vi "Get IRP Waveform.vi"(10 "Channel config":T2={"Voltage channel index"=1, "Shunt channel index"=2, "Shunt resistance"=10.0}, 11 "array":waveform(dbl)[](array[waveform])) -> (1 "Power waveform out":waveform(dbl), 2 "Resistance waveform out":waveform(dbl), 3 "Current waveform out":waveform(dbl), 4 "Channel names":T1)   [LabVIEW 2019]
doc: "This example demonstrates how to acquire a continuous amount of data (Waveform) using the DAQ device's internal clock. It also shows how to synchronize two devices for different device families (E Series, S Series, M Series, X Series, DSA, and SC Express), to simultaneously acquire the data.\n\nFor instructions on how to connect your signals to the DAQ device, refer to your device documentation."
panel:
  # "Get IRP Waveform"
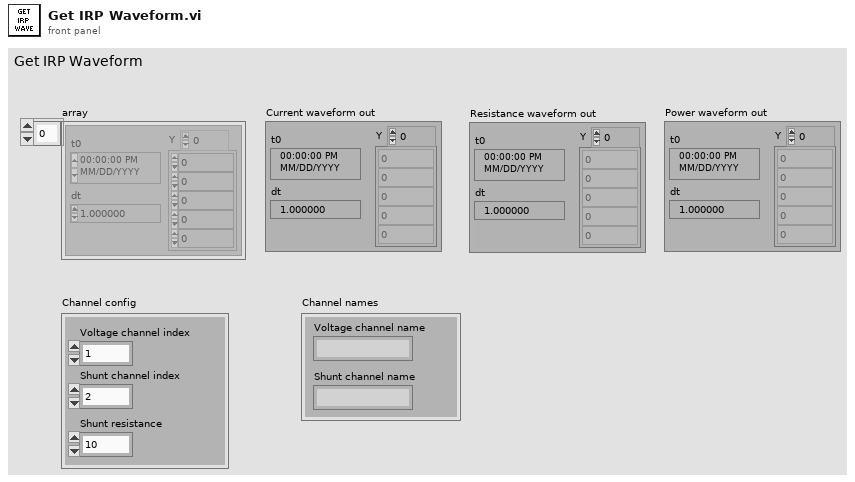
[diagram p1: front panel]
types:
  T1 = cluster{"Voltage channel name":string, "Shunt channel name":string}
  T2 = cluster{"Voltage channel index":i32, "Shunt channel index":i32, "Shunt resistance":dbl}
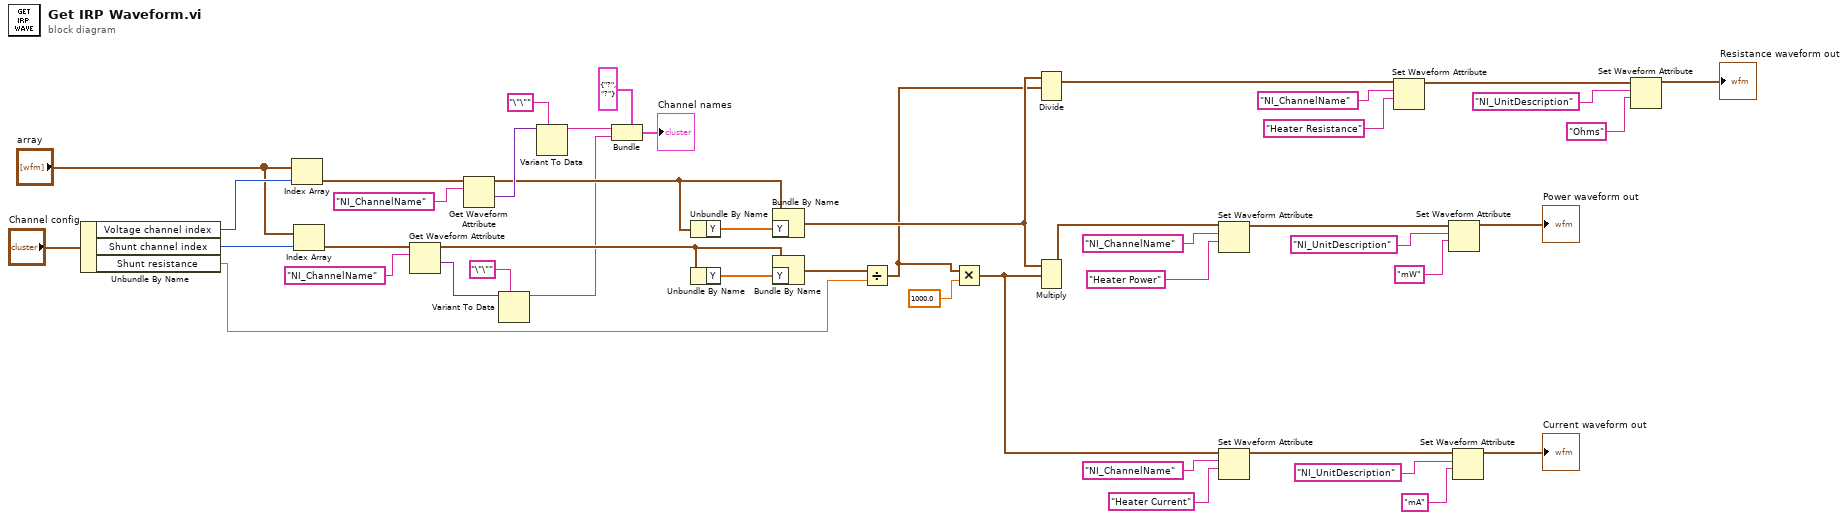
[diagram p0: block diagram]
diagram:
  n1 = Unbundle By Name("Channel config") -> ("Voltage channel index"=w38:i32, "Shunt channel index"=w32:i32, "Shunt resistance"=w1:dbl)
  n2 = Index Array(array="array", index=w38) -> (element=w42:waveform(dbl))
  n3 = Index Array(array="array", index=w32) -> (element=w27:waveform(dbl))
  n4 = Get Waveform Attribute(6:"NI_ChannelName" ("name"), 7:w27) -> (1:w28:variant, 3:w25:waveform(dbl))  [unwired: 2 in, 2 out]
  n5 = Get Waveform Attribute(6:"NI_ChannelName" ("name"), 7:w42) -> (1:w36:variant, 3:w35:waveform(dbl))  [unwired: 2 in, 2 out]
  n6 = Variant To Data(type="\"\"" ("name"), Variant=w28) -> (data=w6:string)  [unwired: 1 in, 1 out]
  n7 = Variant To Data(type="\"\"" ("name"), Variant=w36) -> (data=w7:string)  [unwired: 1 in, 1 out]
  n8 = Bundle(cluster=cluster{"name":string, "name":string} {"name"="?", "name"="?"}, "name"=w7, "name"=w6) -> (→"Channel names":cluster{"name":string, "name":string})
  n9 = Unbundle By Name(w35) -> ("Y"=w34:dbl[])
  n10 = Unbundle By Name(w25) -> ("Y"=w26:dbl[])
  n11 = Bundle By Name(cluster=w35, "Y"=w34) -> (w10:waveform(dbl))
  n12 = Bundle By Name(cluster=w25, "Y"=w26) -> (w9:waveform(dbl))
  n13 = Divide(x=w9, y=w1) -> (x/y=w2:waveform(dbl))
  n14 = Multiply(x=w2, y=1000.0) -> (x*y=w3:waveform(dbl))
  n15 = Divide(1:w2, 2:w10) -> (0:w8:waveform(dbl))  [unwired: 1 in, 1 out]
  n16 = Multiply(1:w3, 2:w10) -> (0:w33:waveform(dbl))  [unwired: 1 in, 1 out]
  n17 = Set Waveform Attribute(5:"Heater Power" ("name"), 6:"NI_ChannelName" ("name"), 7:w33) -> (3:w44:waveform(dbl))  [unwired: 1 in, 2 out]
  n18 = Set Waveform Attribute(5:"Heater Current" ("name"), 6:"NI_ChannelName" ("name"), 7:w3) -> (3:w17:waveform(dbl))  [unwired: 1 in, 2 out]
  n19 = Set Waveform Attribute(5:"Heater Resistance" ("name"), 6:"NI_ChannelName" ("name"), 7:w8) -> (3:w22:waveform(dbl))  [unwired: 1 in, 2 out]
  n20 = Set Waveform Attribute(5:"mW" ("name"), 6:"NI_UnitDescription" ("name"), 7:w44) -> (3:→"Power waveform out":waveform(dbl))  [unwired: 1 in, 2 out]
  n21 = Set Waveform Attribute(5:"mA" ("name"), 6:"NI_UnitDescription" ("name"), 7:w17) -> (3:→"Current waveform out":waveform(dbl))  [unwired: 1 in, 2 out]
  n22 = Set Waveform Attribute(5:"Ohms" ("name"), 6:"NI_UnitDescription" ("name"), 7:w22) -> (3:→"Resistance waveform out":waveform(dbl))  [unwired: 1 in, 2 out]
